vi "MeasureRMS.vi"(10 "Input":T1) -> (1 "Waveform Graph":dynamicdata(graph), 2 "RMS":dbl)   [LabVIEW 2014]
uses:
  <vilib>/Analysis/5stat.llb/RMS (DBL).vi
  <vilib>/Analysis/NI_AALPro.lvlib
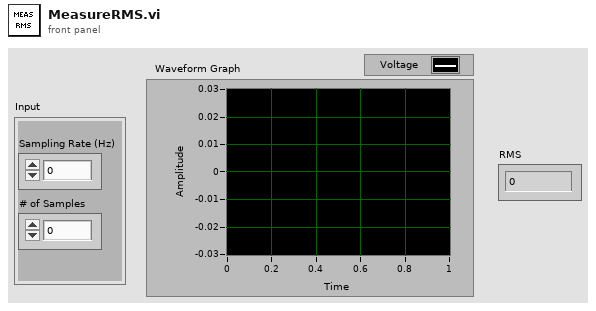
[diagram p1: front panel]
types:
  T1 = cluster{"Sampling Rate (Hz)":dbl, "# of Samples":i64}
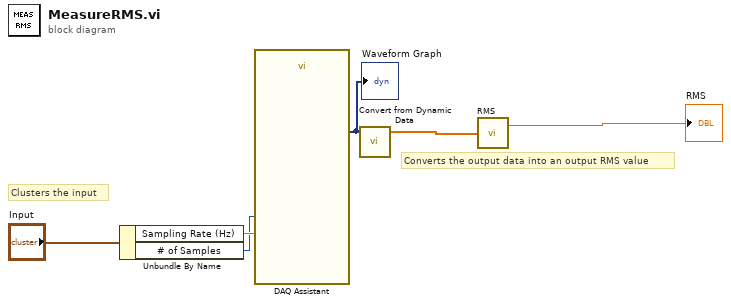
[diagram p0: block diagram]
diagram:
  # "Converts the output data into an output RMS value"
  # "Clusters the input"
  n1 = Unbundle By Name("Input") -> ("Sampling Rate (Hz)"=w2:dbl, "# of Samples"=w1:i64)
  n2 = call "DAQ Assistant"("rate"=w2, "number of samples"=w1) -> ("data"=w6:dynamicdata)  [unwired: 15 in, 2 out]
  "Waveform Graph" <- w6
  n3 = call "Convert from Dynamic Data"("Dynamic Data Type"=w6) -> ("Array"=w5:dbl[])  [unwired: 3 in]
  n4 = call-poly <vilib>:"RMS.vi"("X"=w5) -> ("rms value"=→"RMS":dbl)  [unwired: 1 out]
